vi "Vision Processing.vi"(4 "error in (no error)":errorcluster, 7 "Image Size":T1=enum."320x240") -> ()   [LabVIEW 2018]
doc: "This VI runs in parallel to other tasks. It gets images from the camera, processes them for color or shape and use that information to affect robot behavior."
uses:
  <vilib>/Rock Robotics/WPI/Camera/WPI_CameraImageSize.ctl
  <vilib>/Rock Robotics/WPI/Camera/WPI_CameraWhite Balance Values.ctl
  <vilib>/Rock Robotics/WPI/Camera/WPI_CameraExposure Values.ctl
  <vilib>/Rock Robotics/WPI/Camera/WPI_CameraFrameRate.ctl
  Robot Global Data.vi
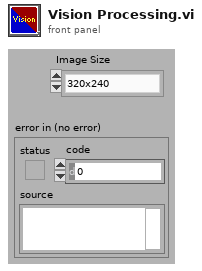
[diagram p1: front panel]
types:
  T1 = typedef "WPI_CameraImageSize.ctl" = enum16{"640x480", "320x240", "160x120", "Custom"}
  T2 = typedef "WPI_CameraFrameRate.ctl" = u32
  T3 = typedef "WPI_CameraExposure Values.ctl" = enum16{"Auto", "Flicker-free 50 Hz", "Flicker-free 60 Hz", "Hold current", "Custom"}
  T4 = typedef "WPI_CameraWhite Balance Values.ctl" = enum16{"Auto", "Fixed indoor", "Fixed outdoor 1", "Fixed outdoor 2", "Fixed fluorescent 1", "Fixed fluorescent 2", "Hold current", "Custom"}
  T5 = typedef "Image Type" = u32
  T6 = typedef "WPI_CameraDevRef.ctl" = cluster{"Camera Address":string, "CameraStatus":errorcluster}
  T7 = typedef "IMAQ Image.ctl" = refnum<image>
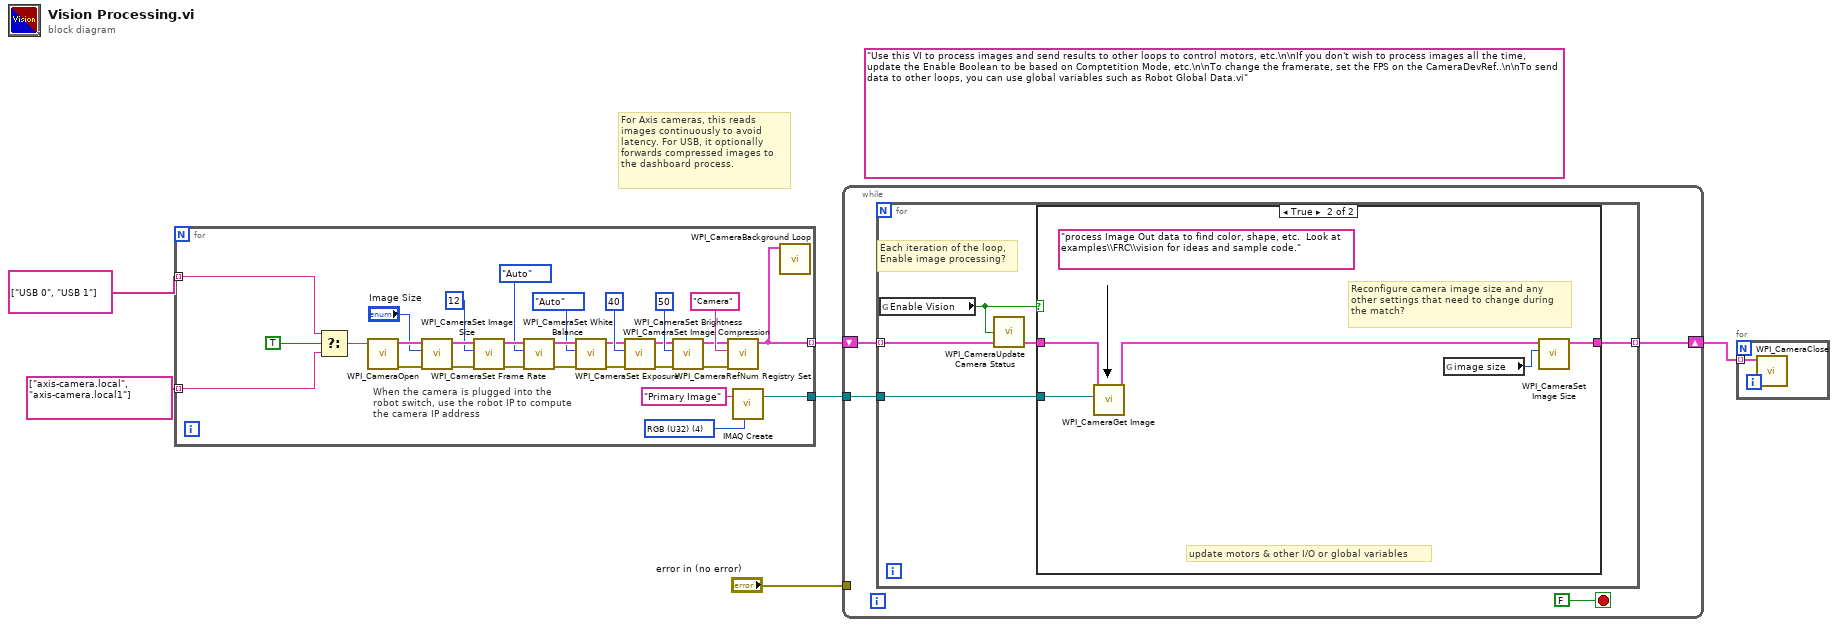
[diagram p0: block diagram]
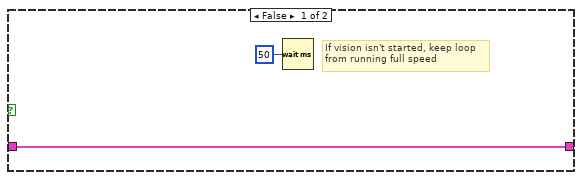
[diagram p2: hidden frame]
diagram:
  (unwired) "Use this VI to process images and send results to other loops to control motors, etc.\n\nIf you don't wish to process images all the time, update the Enable Boolean to be based on Comptetition Mode, etc.\n\nTo change the framerate, set the FPS on the CameraDevRef..\n\nTo send data to other loops, you can use global variables such as Robot Global Data.vi"
  # "For Axis cameras, this reads\nimages continuously to avoid\nlatency. For USB, it optionally\nforwards compressed images to\nthe dashboard process."
  n1 = for {
    tunnel: [w33] -> w6
    tunnel: [w12] -> w5 mode=indexing
    tunnel: string[] ["USB 0", "USB 1"] ("format string") -> [w8] mode=indexing
    tunnel: string[] ["axis-camera.local", "axis-camera.local1"] ("format string") -> [w7] mode=indexing
    w35 = T5 4 items=["Grayscale (U8)", "Grayscale (I16)", "Grayscale (SGL)", "Complex (CSG)", "RGB (U32)", "HSL (U32)", "RGB (U64)"] ("Image Type")
    # "When the camera is plugged into the\nrobot switch, use the robot IP to compute\nthe camera IP address"
    n2 = Select(t=w8, s=TRUE ("dot notation? (F)"), f=w7) -> (s? t:f=w9:string)
    n3 = call <vilib>:"WPI_CameraOpen.vi"("Camera Address"=w9) -> ("error out"=w23:errorcluster, "CameraDevRef"=w24:T6)  [unwired: 1 in, 8 out]
    n4 = call <vilib>:"WPI_CameraSet Image Size.vi"("error in (no error)"=w23, "Image Size"="Image Size", "CameraDevRef"=w24) -> ("error out"=w22:errorcluster, "CameraDevRef Out"=w25:T6)  [unwired: 1 in, 6 out]
    n5 = call <vilib>:"WPI_CameraSet Frame Rate.vi"("error in (no error)"=w22, "Frame Rate (fps)"=T2 12, "CameraDevRef"=w25) -> ("error out"=w21:errorcluster, "CameraDevRef Out"=w27:T6)  [unwired: 7 out]
    n6 = call <vilib>:"WPI_CameraSet White Balance.vi"("error in (no error)"=w21, "White Balance"=WPI_CameraWhite_Balance_Values."Auto", "CameraDevRef"=w27) -> ("error out"=w20:errorcluster, "CameraDevRef Out"=w26:T6)  [unwired: 1 in, 6 out]
    n7 = call <vilib>:"WPI_CameraSet Exposure.vi"("error in (no error)"=w20, "Exposure"=WPI_CameraExposure_Values."Auto", "CameraDevRef"=w26) -> ("error out"=w19:errorcluster, "CameraDevRef Out"=w29:T6)  [unwired: 1 in, 6 out]
    n8 = call <vilib>:"WPI_CameraSet Image Compression.vi"("error in (no error)"=w19, "Compression"=40, "CameraDevRef"=w29) -> ("error out"=w18:errorcluster, "CameraDevRef Out"=w28:T6)  [unwired: 7 out]
    n9 = call <vilib>:"WPI_CameraSet Brightness.vi"("error in (no error)"=w18, "Brightness"=50, "CameraDevRef"=w28) -> ("error out"=w16:errorcluster, "CameraDevRef Out"=w17:T6)  [unwired: 1 in, 6 out]
    n10 = call <vilib>:"WPI_CameraRefNum Registry Set.vi"("error in (no error)"=w16, "refnum name"="Camera", "CameraDevRef"=w17) -> ("CameraDevRef"=w12:T6)  [unwired: 1 in, 7 out]
    n11 = call "IMAQ Create"("Image Name"="Primary Image", "Image Type"=w35) -> ("New Image"=w33:T7)  [unwired: 2 in, 2 out]
    n12 = call <vilib>:"WPI_CameraBackground Loop.vi"("CameraDevRef"=w12) -> ()  [unwired: 11 in]
  }
  n13 = while {
    shift-right: [w38] -> w4
    shift-left: w5 -> [w36]
    tunnel: w6 -> [w37]
    tunnel: "error in (no error)" -> [_]
    stop <- FALSE stop-if-true
    n14 = for {
      tunnel: w37 -> [w43]
      tunnel: w36 -> [w42] mode=indexing
      tunnel: [w44] -> w38 mode=indexing
      # "Each iteration of the loop,\nEnable image processing?"
      n15 = global read "Robot Global Data.vi" "Enable Vision"() -> (w40:bool)
      n16 = call <vilib>:"WPI_CameraUpdate Camera Status.vi"("CameraDevRef In"=w42, "Enable Vision"=w40) -> ("CameraDevRef Out"=w41:T6)  [unwired: 3 in]
      n17 = case shown="True" w40 {
        tunnel: w43 -> [_ w50]
        tunnel: [w46 w51] -> w44
        tunnel: w41 -> [w46 w48]
        frame False {
          # "If vision isn't started, keep loop\nfrom running full speed"
          n18 = Wait (ms)(milliseconds to wait=u32 50) -> ()  [unwired: 1 out]
        }
        frame True {
          (unwired) "process Image Out data to find color, shape, etc.  Look at examples\\FRC\\vision for ideas and sample code."
          # "update motors & other I/O or global variables"
          # "Reconfigure camera image size and any\nother settings that need to change during\nthe match?"
          n19 = call <vilib>:"WPI_CameraGet Image.vi"("Image"=w50, "CameraDevRef"=w48) -> ("CameraDevRef Out"=w47:T6)  [unwired: 1 in, 8 out]
          n20 = global read "Robot Global Data.vi" "image size"() -> (w49:T1)
          n21 = call <vilib>:"WPI_CameraSet Image Size.vi"("Image Size"=w49, "CameraDevRef"=w47) -> ("CameraDevRef Out"=w51:T6)  [unwired: 2 in, 7 out]
        }
      }
    }
  }
  n22 = for {
    tunnel: w4 -> [w52] mode=indexing
    n23 = call <vilib>:"WPI_CameraClose.vi"("CameraDevRef"=w52) -> ()  [unwired: 1 in, 10 out]
  }
